vi "FlatToRichnidaqmx_grpc_CreateDOChanRequest.vi"(5 "OutputClusterType":T1, 11 "InputCluster":T3) -> (3 "OutputCluster":T1)   [LabVIEW 2021, in "NI DAQmx_server.lvlib"]
uses:
  NI DAQmx_server.lvlib
  nidaqmx_grpc_CreateDOChanRequest_Flat.ctl
  nidevice_grpc_Session_Flat.ctl
  nidaqmx_grpc_LineGrouping.ctl
  nidaqmx_grpc_CreateDOChanRequest.ctl
  nidevice_grpc_Session_session/nidevice_grpc_Session_session.lvclass
  nidaqmx_grpc_CreateDOChanRequest_line_grouping_enum/nidaqmx_grpc_CreateDOChanRequest_line_grouping_enum.lvclass
  nidevice_grpc_Session.ctl
  nidevice_grpc_Session_session/nidevice_grpc_Session_session.lvclass/nidevice_grpc_Session_session.ctl
  nidaqmx_grpc_CreateDOChanRequest_line_grouping_enum/nidaqmx_grpc_CreateDOChanRequest_line_grouping_enum.lvclass/nidaqmx_grpc_CreateDOChanRequest_line_grouping_enum.ctl
  nidevice_grpc_Session_session/Setname.vi
  nidevice_grpc_Session_session/Setid.vi
  nidevice_grpc_Session_session/GetFieldFromProtobufIndexnidevice_grpc_Session_session.vi
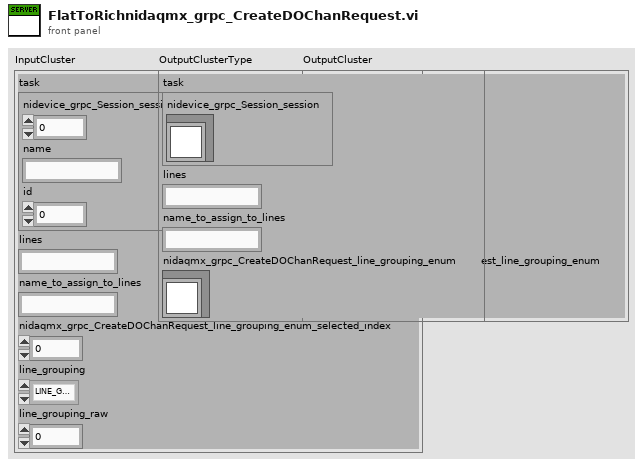
[diagram p1: front panel]
types:
  T1 = typedef "NI DAQmx_server.lvlib/nidaqmx_grpc_CreateDOChanRequest.ctl" = cluster{"task":T2, "lines":string, "name_to_assign_to_lines":string, "nidaqmx_grpc_CreateDOChanRequest_line_grouping_enum":refnum<class "nidaqmx_grpc_CreateDOChanRequest_line_grouping_enum.lvclass">}
  T2 = typedef "NI DAQmx_server.lvlib/nidevice_grpc_Session.ctl" = cluster{"nidevice_grpc_Session_session":refnum<class "nidevice_grpc_Session_session.lvclass">}
  T3 = typedef "NI DAQmx_server.lvlib/nidaqmx_grpc_CreateDOChanRequest_Flat.ctl" = cluster{"task":T4, "lines":string, "name_to_assign_to_lines":string, "nidaqmx_grpc_CreateDOChanRequest_line_grouping_enum_selected_index":i32, "line_grouping":T5, "line_grouping_raw":i32}
  T4 = typedef "NI DAQmx_server.lvlib/nidevice_grpc_Session_Flat.ctl" = cluster{"nidevice_grpc_Session_session_selected_index":i32, "name":string, "id":u32}
  T5 = typedef "NI DAQmx_server.lvlib/nidaqmx_grpc_LineGrouping.ctl" = enum32{"LINE_GROUPING_CHAN_PER_LINE", "LINE_GROUPING_CHAN_FOR_ALL_LINES"}
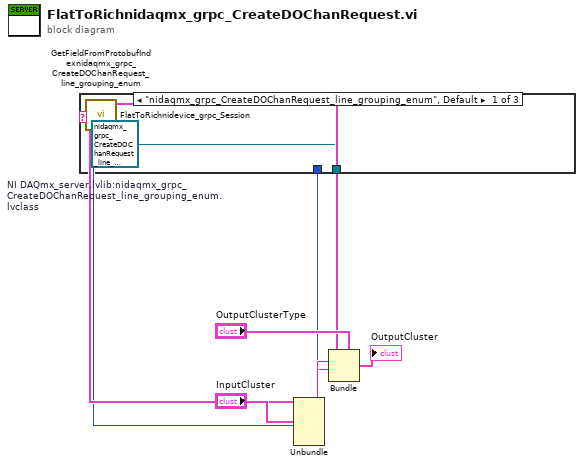
[diagram p0: block diagram]
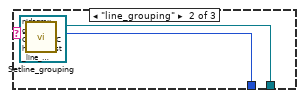
[diagram p2: hidden frame]
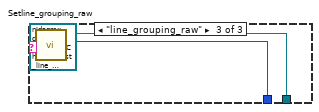
[diagram p3: hidden frame]
diagram:
  n1 = Unbundle "Unbundle"("InputCluster") -> ("task"=w9:T4, "lines"=w7:string, "name_to_assign_to_lines"=w6:string, "nidaqmx_grpc_CreateDOChanRequest_line_grouping_enum_selected_index"=w5:i32, "line_grouping"=w2:T5, "line_grouping_raw"=w1:i32)
  n2 = call "GetFieldFromProtobufIndexnidaqmx_grpc_CreateDOChanRequest_line_grouping_enum.vi"("protobuf index"=w5) -> ("oneof field name"=w4:string)
  n3 = case "nidaqmx_grpc_CreateDOChanRequest_line_grouping_enum" shown="\"nidaqmx_grpc_CreateDOChanRequest_line_grouping_enum\", Default" w4 {
    tunnel: [w13 w15 w18] -> w3
    tunnel: w2 -> [_ w16 _]
    tunnel: w1 -> [_ _ w19]
    frame "nidaqmx_grpc_CreateDOChanRequest_line_grouping_enum", Default {
      w13 = refnum<class "nidaqmx_grpc_CreateDOChanRequest_line_grouping_enum.lvclass"> refnum  # NI DAQmx_server.lvlib:nidaqmx_grpc_CreateDOChanRequest_line_grouping_enum.lvclass
    }
    frame "line_grouping" {
      n4 = call "Setline_grouping.vi"("Set_Val"=w16, "OneOfTemplate in"=refnum<class "nidaqmx_grpc_CreateDOChanRequest_line_grouping_enum.lvclass"> refnum) -> ("OneOfTemplate out"=w15:refnum<class "nidaqmx_grpc_CreateDOChanRequest_line_grouping_enum.lvclass">)  [unwired: 8 in, 1 out]
    }
    frame "line_grouping_raw" {
      n5 = call "Setline_grouping_raw.vi"("Set_Val"=w19, "OneOfTemplate in"=refnum<class "nidaqmx_grpc_CreateDOChanRequest_line_grouping_enum.lvclass"> refnum) -> ("OneOfTemplate out"=w18:refnum<class "nidaqmx_grpc_CreateDOChanRequest_line_grouping_enum.lvclass">)  [unwired: 8 in, 1 out]
    }
  }
  n6 = call "FlatToRichnidevice_grpc_Session.vi"("InputCluster"=w9) -> ("OutputCluster"=w8:T2)  [unwired: 10 in]
  n7 = Bundle "Bundle"(cluster="OutputClusterType", "task"=w8, "lines"=w7, "name_to_assign_to_lines"=w6, "nidaqmx_grpc_CreateDOChanRequest_line_grouping_enum"=w3) -> (→"OutputCluster":T1)
